vi "get values for workspace.vi"(9 "Arr Refnum":refnum<vi>) -> (3 "appended array":dbl[][](array[numeric]), 4 "element":string, 5 "String":string)   [LabVIEW 2016]
uses:
  controls/data control cluster.ctl
panel:
  out "Cycle data by position":dbl[][][](array[numeric])
  out "t":i32
  out "index of element":i32
  out "DATA CLUSTER out":T1
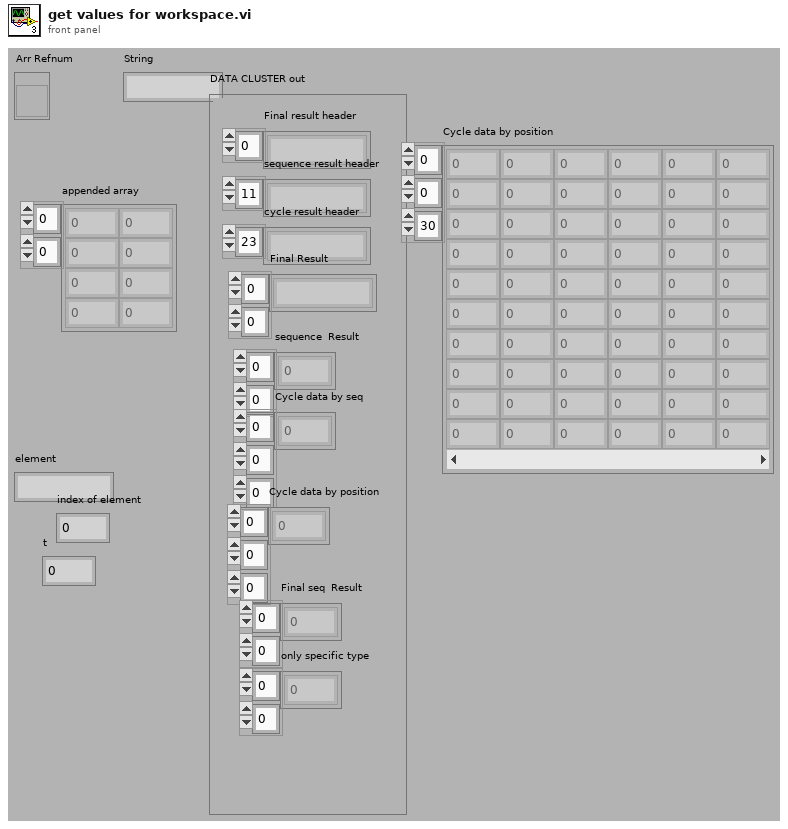
[diagram p1: front panel]
types:
  T1 = typedef "data control cluster.ctl" = cluster{"Final result header":string[], "sequence result header":string[], "cycle result header ":string[], "Final Result":string[][], "sequence  Result":dbl[][], "Cycle data by seq":dbl[][][], "Cycle data by position":dbl[][][], "Final seq  Result":dbl[][], "only specific type":dbl[][]}
  T2 = typedef "cycle results control.ctl" = cluster{"sample info":string[][], "cycle results labels":string[], "cycle results dbl":dbl[][]}
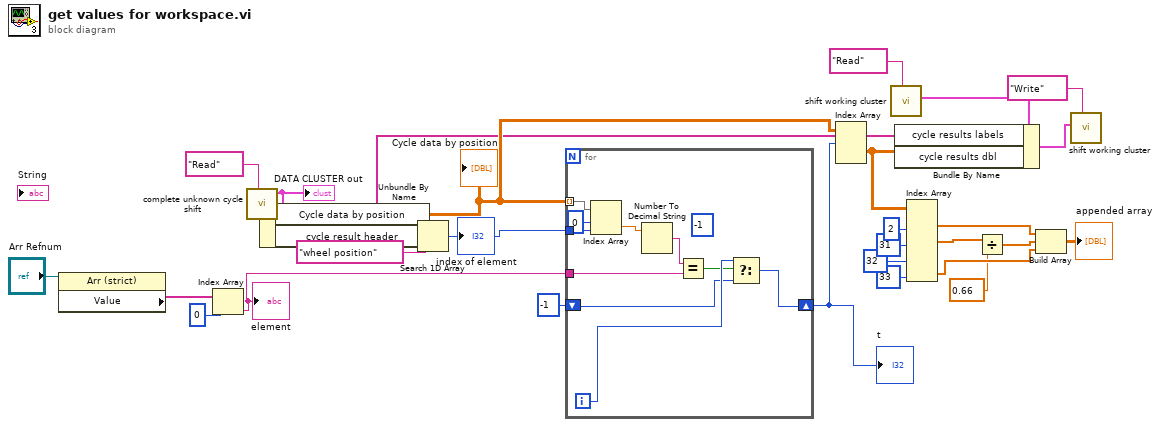
[diagram p0: block diagram]
diagram:
  n1 = property on="Property Node" class="Arr (strict)"(reference="Arr Refnum") -> ("Value"=w25:string[])  [unwired: 1 in, 2 out]
  n2 = Index Array(array=w25, index=0) -> (element=w19:string)
  "element" <- w19
  n3 = call "complete unknown cycle shift.vi"("read write shift"="Read") -> ("DATA CLUSTER out"=w23:T1)  [unwired: 9 in, 1 out]
  "DATA CLUSTER out" <- w23
  n4 = Unbundle By Name(w23) -> ("Cycle data by position"=w16:dbl[][][], "cycle result header"=w14:string[])
  "Cycle data by position" <- w16
  n5 = Search 1D Array(1D array=w14, element="wheel position") -> (index of element=w21:i32)  [unwired: 1 in]
  "index of element" <- w21
  n6 = for {
    tunnel: w16 -> [w37] mode=indexing
    tunnel: w21 -> [w36]
    tunnel: w19 -> [w34]
    shift-right: [w33] -> w15
    shift-left: -1 ("t") -> [w31]
    i -> [w32]
    (unwired) -1 ("t")
    n7 = Index Array(array=w37, index (row)=0 ("disabled index (row)"), index (col)=w36) -> (element=w29:dbl)
    n8 = Number To Decimal String(number=w29) -> (decimal integer string=w35:string)  [unwired: 1 in]
    n9 = Equal?(x=w35, y=w34) -> (x = y?=w30:bool)
    n10 = Select(t=w32, s=w30, f=w31) -> (s? t:f=w33:i32)
  }
  "t" <- w15
  n11 = Index Array(array=w16, index (dim 0)=w15) -> (element=w11:dbl[][])  [unwired: 2 in]
  n12 = call "shift working cluster.vi"("read write shift"="Read") -> ("cycle results cluster out"=w18:T2)  [unwired: 9 in, 1 out]
  n13 = Bundle By Name(cluster=w18, "cycle results labels"=w14, "cycle results dbl"=w11) -> (w12:T2)
  n14 = Index Array(array=w11, index (col) #1=2 ("disabled index (col)"), index (col) #2=31 ("index (col)"), index (col) #3=32 ("index (col)"), index (col) #4=33 ("index (col)")) -> (element #1=w7:dbl[], element #2=w5:dbl[], element #4=w2:dbl[])  [unwired: 4 in, 1 out]
  n15 = Divide(x=w5, y=0.66 ("Numeric")) -> (x/y=w4:dbl[])
  n16 = Build Array(w7, w4, w2) -> (→"appended array":dbl[][])
  n17 = call "shift working cluster.vi"("read write shift"="Write", "cycle results cluster In"=w12) -> ()  [unwired: 8 in, 2 out]
